vi "SerialInit.vi"(8 "error in (no error)":errorcluster, 10 "PID":i32, 11 "IPC":i32) -> (0 "error out":errorcluster)   [LabVIEW 2013, in "Advanced Plotting Toolkit.lvlib"]
uses:
  Advanced Plotting Toolkit.lvlib
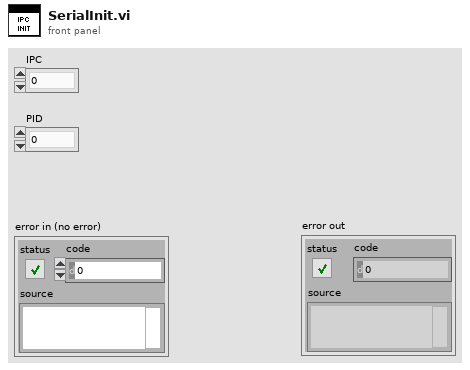
[diagram p1: front panel]
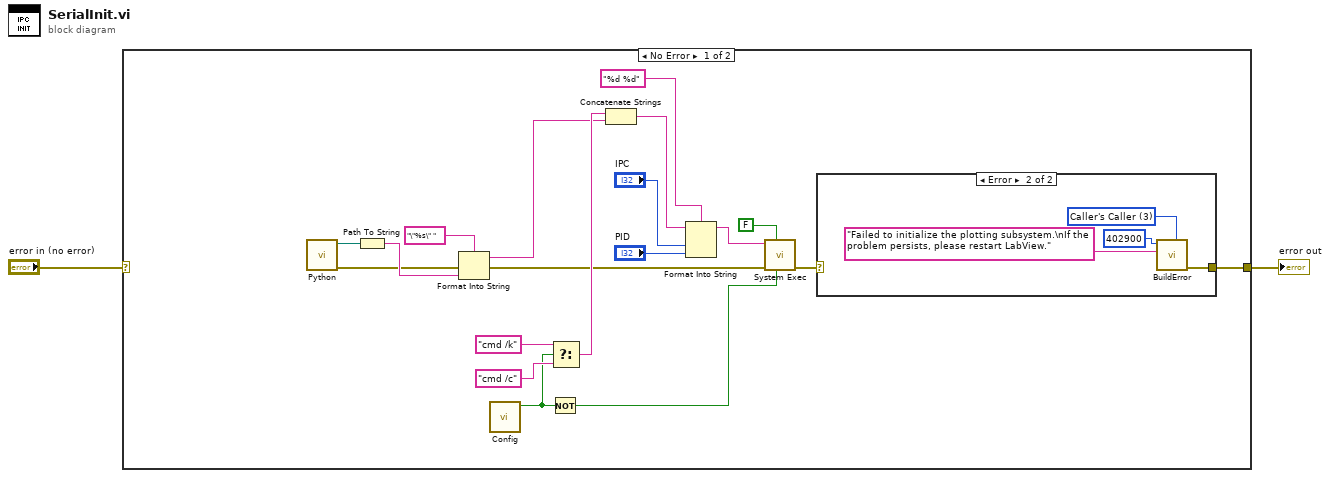
[diagram p0: block diagram]
diagram:
  n1 = case shown="No Error" "error in (no error)" {
    selector: "error in (no error)" -> [_ w27]
    tunnel: [w21 w27] -> w1
    frame No Error {
      n2 = call "Python.vi"() -> ("error out"=w3:errorcluster, "BinCache"=w6:path)  [unwired: 10 in]
      n3 = Path To String(path=w6) -> (string=w5:string)
      n4 = Format Into String(format string="\"%s\" ", error in=w3, w5) -> (resulting string=w10:string, error out=w9:errorcluster)  [unwired: 1 in]
      n5 = call "Config.vi"() -> ("Show Console"=w11:bool)  [unwired: 11 in]
      n6 = Not(x=w11) -> (.not. x?=w12:bool)
      n7 = Select(t="cmd /k", s=w11, f="cmd /c") -> (s? t:f=w14:string)
      n8 = Concatenate Strings(w14, w10) -> (w13:string)
      n9 = Format Into String(format string="%d %d", initial string=w13, "IPC", "PID") -> (resulting string=w18:string)  [unwired: 1 in, 1 out]
      n10 = call <vilib>:"System Exec.vi"("run minimized? (F)"=w12, "wait until completion? (T)"=FALSE, "error in (no error)"=w9, "command line"=w18) -> ("error out"=w8:errorcluster)  [unwired: 4 in, 3 out]
      n11 = case shown="Error" w8 {
        selector: w8 -> [w22 _]
        tunnel: [w22 w24] -> w21
        frame No Error {
        }
        frame Error {
          w23 = u16 3 items=["Caller"=2, "Caller's Caller"=3] ("Source")
          n12 = call "BuildError.vi"(5:"Source"=w23, 10:"Source"="Failed to initialize the plotting subsystem.\nIf the problem persists, please restart LabView." ("error message (\"\")"), "Code"=402900 ("error code (0)")) -> ("error out"=w24:errorcluster)  [unwired: 8 in]
        }
      }
    }
    frame Error {
    }
  }
  "error out" <- w1
